vi "XML - Get XML file name.vi"(10 "CD Template":refnum<class "NIVS_CD Template.lvclass">, 11 "CD Name":string) -> (3 "XML file name":string)   [LabVIEW 2015, in "NIVS_Consolidated_CDW_MetaDataObj.lvclass"]
doc: "Determines the file name of the XML file based on the name and execution mode of the custom device."
uses:
  NIVS_Consolidated_CDW_MetaDataObj.lvclass
  Template Classes/NIVS_CD Template/NIVS_CD Template.lvclass
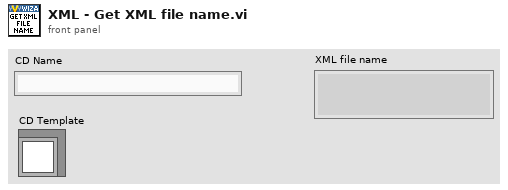
[diagram p1: front panel]
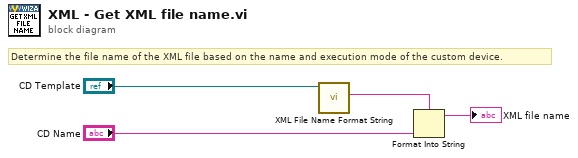
[diagram p0: block diagram]
diagram:
  # "Determine the file name of the XML file based on the name and execution mode of the custom device."
  n1 = call-dynamic "XML File Name Format String.vi"("CD Template"="CD Template") -> ("XML File Name Format String"=w2:string)  [unwired: 10 in]
  n2 = Format Into String(format string=w2, "CD Name") -> (resulting string=→"XML file name":string)  [unwired: 2 in, 1 out]
